vi "Error In (Lux).vi"() -> ()   [LabVIEW 2015]
panel:
  in  "Error In":errorcluster
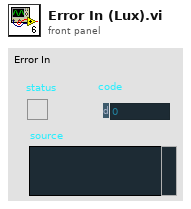
[diagram p1: front panel]
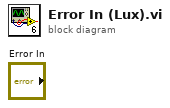
[diagram p0: block diagram]
diagram:
